vi "Delta.vi"(0 "currentValue":dbl, 1 "delta":dbl) -> (7 "triggerEvent":bool)   [LabVIEW 2015]
panel:
  out "previousValue":dbl
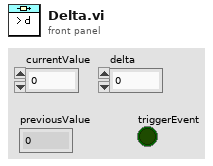
[diagram p1: front panel]
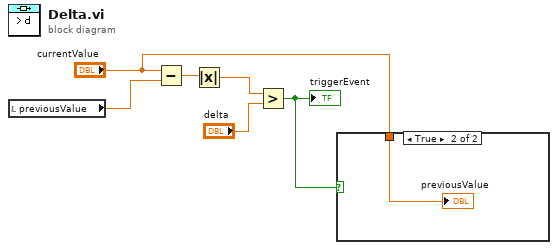
[diagram p0: block diagram]
diagram:
  n1 = local read "previousValue"() -> (w1:dbl)
  n2 = Subtract(x="currentValue", y=w1) -> (x-y=w5:dbl)
  n3 = Absolute Value(x=w5) -> (abs(x)=w4:dbl)
  n4 = Greater?(x=w4, y="delta") -> (0:w3:bool)
  "triggerEvent" <- w3
  n5 = case shown="True" w3 {
    tunnel: "currentValue" -> [_ w7]
    frame False {
    }
    frame True {
      "previousValue" <- w7
    }
  }
